vi "OccupancyGridWithAStar.vi"() -> ()   [LabVIEW 2019]
uses:
  <vilib>/Analysis/6fits.llb/nD B-Spline Fit.vi
  <vilib>/robotics/Navigation/shared/WorldMap/OccupancyGridWorldMap/NI_Robotics_OccupancyGridWorldMap.lvclass
  <vilib>/Analysis/NI_AALPro.lvlib
panel:
  out "Trajectory Plot":cluster{dbl[], dbl[]}[](graph)
  out "Intensity Graph 2":dbl[][](graph) caption="Intensity Graph"
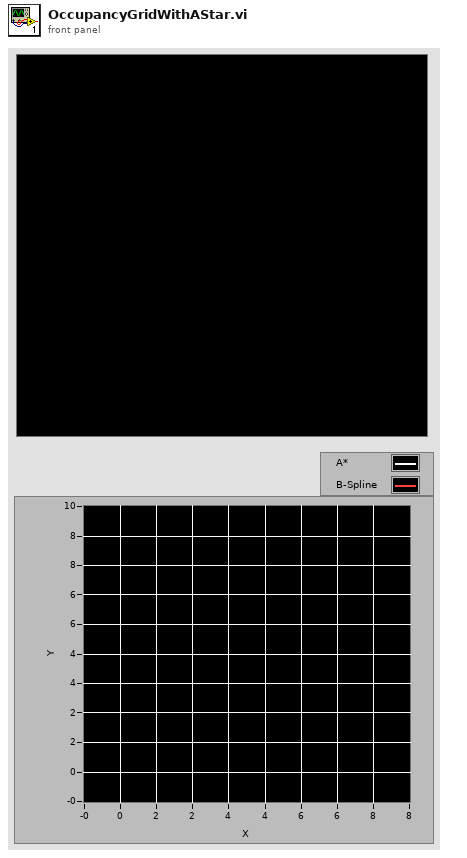
[diagram p1: front panel]
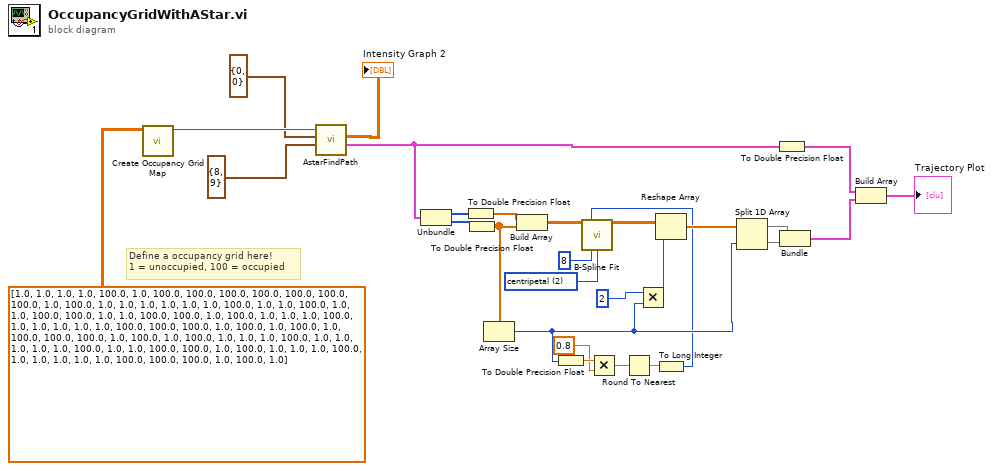
[diagram p0: block diagram]
diagram:
  w18 = u16 2 items=["equally spaced", "chord length", "centripetal"] ("parameter selection")
  # "Define a occupancy grid here!\n1 = unoccupied, 100 = occupied"
  n1 = call <vilib>:"Create Occupancy Grid Map.vi"("occupancy grid"=dbl[][] [[1.0, 1.0, 1.0, 1.0, 100.0, 1.0, 100.0, 100.0, 100.0, 100.0], [100.0, 100.0, 100.0, 1.0, 100.0, 1.0, 1.0, 1.0, 1.0, 1.0], [1.0, 100.0, 1.0, 1.0, 100.0, 1.0, 1.0, 100.0, 100.0, 1.0], [1.0, 100.0, 100.0, 1.0, 100.0, 1.0, 1.0, 1.0, 100.0, 1.0], [1.0, 1.0, 1.0, 1.0, 100.0, 100.0, 100.0, 1.0, 100.0, 1.0], [100.0, 1.0, 100.0, 100.0, 100.0, 1.0, 100.0, 1.0, 100.0, 1.0], [1.0, 1.0, 100.0, 1.0, 1.0, 1.0, 1.0, 1.0, 100.0, 1.0], [1.0, 100.0, 100.0, 1.0, 100.0, 1.0, 1.0, 1.0, 100.0, 1.0], [1.0, 1.0, 1.0, 1.0, 100.0, 100.0, 100.0, 1.0, 100.0, 1.0]]) -> ("map reference out"=w27:refnum<data-value>)  [unwired: 9 in, 1 out]
  n2 = call "AstarFindPath.vi"("goal node"=cluster{"X":i32, "Y":i32} {"X"=8, "Y"=9}, "start node"=cluster{"X":i32, "Y":i32} {"X"=0, "Y"=0}, "map reference in"=w27) -> ("Planned Path"=w13:cluster{i32[], i32[]}, "intensity values"=→"Intensity Graph 2":dbl[][])  [unwired: 5 in, 2 out]
  n3 = Unbundle(w13) -> (w23:i32[], w22:i32[])
  n4 = To Double Precision Float(number=w23) -> (double precision float=w21:dbl[])
  n5 = To Double Precision Float(number=w22) -> (double precision float=w9:dbl[])
  n6 = Array Size(array=w9) -> (size(s)=w6:i32)
  n7 = Build Array(w21, w9) -> (w20:dbl[][])
  n8 = To Double Precision Float(number=w6) -> (double precision float=w3:dbl)
  n9 = Multiply(x=w3, y=0.8) -> (x*y=w1:dbl)
  n10 = Round To Nearest(number=w1) -> (nearest integer value=w5:dbl)
  n11 = Multiply(x=2, y=w6) -> (x*y=w8:i32)
  n12 = To Long Integer(number=w5) -> (32bit integer=w4:i32)
  n13 = call-poly <vilib>:"B-Spline Fit.vi"("Data"=w20, "# of control points"=w4, "degree"=8, "parameter selection"=w18) -> ("Best BSpline Fit"=w17:dbl[][])  [unwired: 9 in, 2 out]
  n14 = Reshape Array(w17, w8) -> (w16:dbl[])
  n15 = Split 1D Array(array=w16, index=w6) -> (first subarray=w15:dbl[], second subarray=w14:dbl[])
  n16 = To Double Precision Float(number=w13) -> (double precision float=w12:cluster{dbl[], dbl[]})
  n17 = Bundle(w15, w14) -> (w11:cluster{dbl[], dbl[]})  [unwired: 1 in]
  n18 = Build Array(w12, w11) -> (→"Trajectory Plot":cluster{dbl[], dbl[]}[])
